vi "read burron.vi"() -> ()   [LabVIEW 2017]
panel:
  in  "GPIO":string(combo)
  out "LED indicator":string="LED OFF"
  out "button state":string="LED is turned on"
  out "error out 2":errorcluster
  in  "stop":bool
  out "error out":errorcluster
  in  "mode (standard)":T1(ring)
  in  "bytes to read":i32=1 min=1
  out "data out":string
  in  "Send Button":bool
  in  "Port":u16
  in  "address":string
  in  "data in":string
  out "bytes written":i32
  in  "stop 1":bool
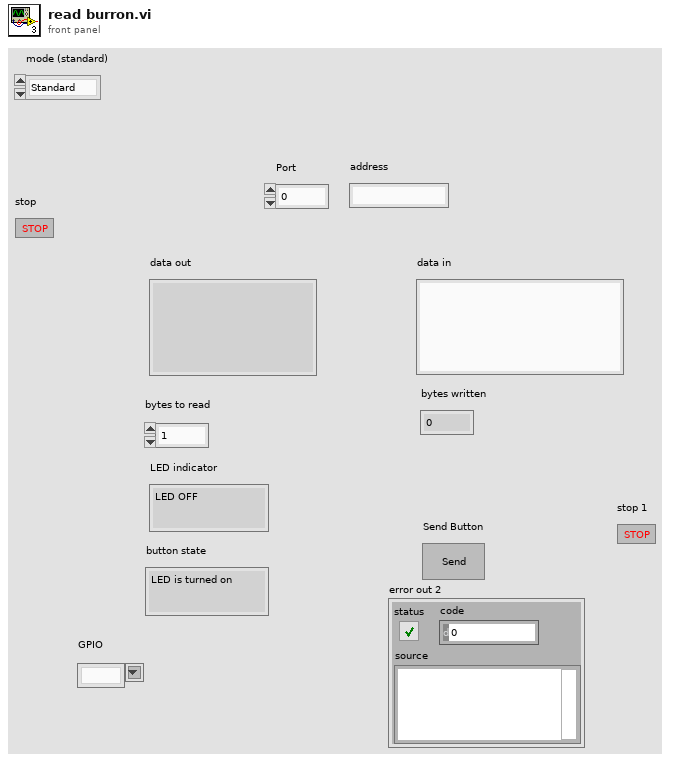
[diagram p1: front panel]
types:
  T1 = enum16{"Standard", "Buffered", "CRLF", "Immediate"}
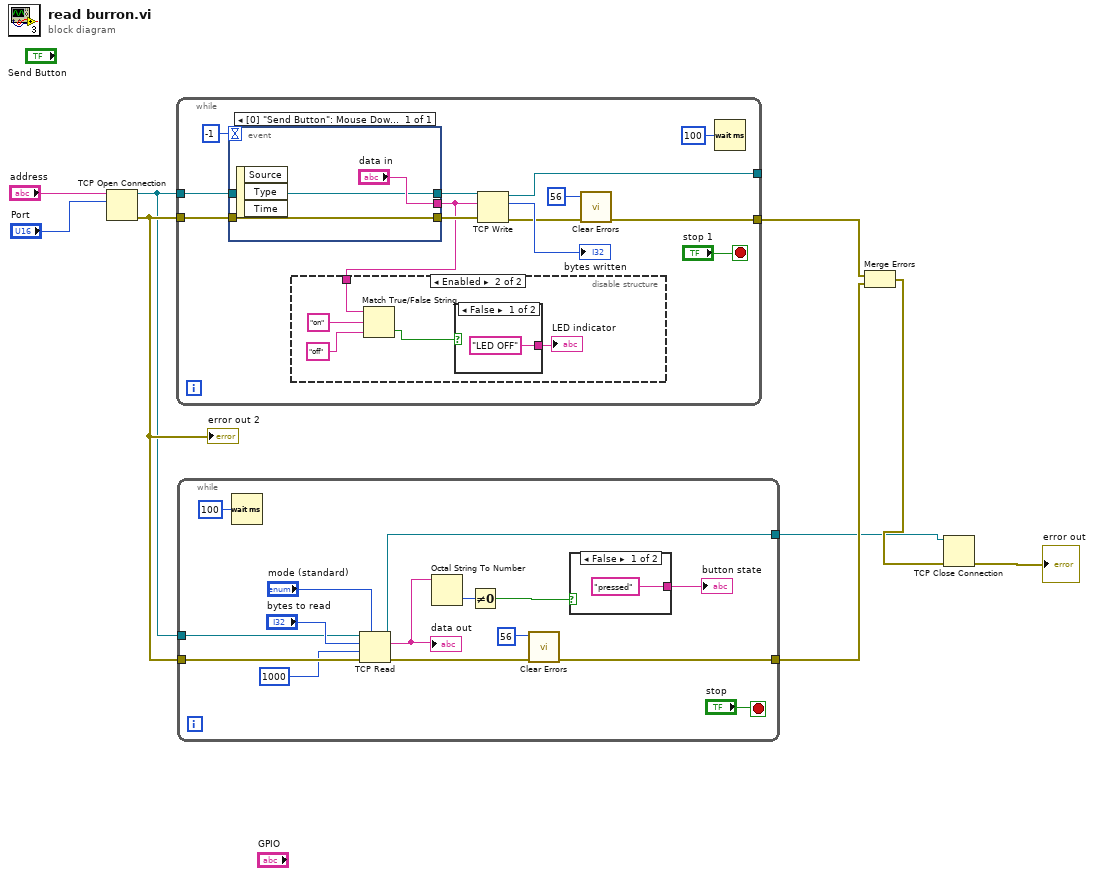
[diagram p0: block diagram]
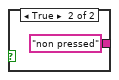
[diagram p2: hidden frame]
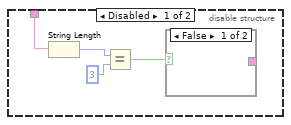
[diagram p3: hidden frame]
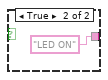
[diagram p4: hidden frame]
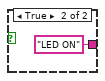
[diagram p5: hidden frame]
diagram:
  n1 = TCP Open Connection(address="address", remote port or service name="Port") -> (connection ID=w1:refnum<k5>, error out=w2:errorcluster)  [unwired: 3 in]
  "error out 2" <- w2
  n2 = while {
    tunnel: w1 -> [w12]
    tunnel: [w22] -> _
    tunnel: w2 -> [w15]
    tunnel: [w16] -> w7
    stop <- "stop 1" stop-if-true
    n3 = event shown="[0] \"Send Button\": Mouse Down;  Timeout" {
      selector: _ -> [_]
      dyn-events: _ -> [_]
      timeout: -1 -> [_]
      tunnel: ["data in"] -> w10
      tunnel: w15 -> [w36]
      tunnel: [w36] -> w14
      tunnel: [w35] -> w13
      tunnel: w12 -> [w35]
      event "Send Button": Mouse Down; Timeout {
        n4 = event-data() -> ()  [unwired: 1 in, 3 out]
      }
    }
    n5 = disable-structure shown="Enabled" {
      disable-tunnel: w10 -> [w26 w31]
      frame Disabled {
        n6 = String Length(string=w26) -> (length=w25:i32)
        n7 = Equal?(x=w25, y=3) -> (x = y?=w23:bool)
        n8 = case shown="False" w23 {
          tunnel: [_ "LED ON"] -> _
          frame False {
          }
          frame True {
          }
        }
      }
      frame Enabled {
        n9 = Match True/False String(2:"off" ("false string"), 3:"on" ("true string"), 4:w31) -> (0:w28:bool)  [unwired: 1 out]
        n10 = case shown="False" w28 {
          tunnel: ["LED OFF" "LED ON"] -> w32
          frame False {
          }
          frame True {
          }
        }
        "LED indicator" <- w32
      }
    }
    n11 = TCP Write(connection ID=w13, data in=w10, error in (no error)=w14) -> (connection ID out=w22:refnum<k5>, bytes written=→"bytes written":i32, error out=w17:errorcluster)  [unwired: 1 in]
    n12 = call <vilib>:"Clear Errors.vi"("error in (no error)"=w17, "specific error code to clear (0: all)"=56) -> ("error out"=w16:errorcluster)  [unwired: 4 in, 1 out]
    n13 = Wait (ms)(milliseconds to wait=u32 100) -> ()  [unwired: 1 out]
  }
  n14 = while {
    tunnel: [w48] -> w4
    tunnel: [w47] -> w3
    tunnel: w2 -> [w46]
    tunnel: w1 -> [w45]
    stop <- "stop" stop-if-true
    n15 = Wait (ms)(milliseconds to wait=u32 100) -> ()  [unwired: 1 out]
    n16 = TCP Read(connection ID=w45, bytes to read="bytes to read", error in (no error)=w46, 7:"mode (standard)", 9:1000 ("timeout ms (25000)")) -> (connection ID out=w47:refnum<k5>, data out=w39:string, error out=w51:errorcluster)
    "data out" <- w39
    n17 = Octal String To Number(4:w39) -> (0:w41:u32)  [unwired: 2 in, 1 out]
    n18 = Not Equal To 0?(x=w41) -> (x != 0?=w42:bool)
    n19 = call <vilib>:"Clear Errors.vi"("error in (no error)"=w51, "specific error code to clear (0: all)"=56) -> ("error out"=w48:errorcluster)  [unwired: 4 in, 1 out]
    n20 = case shown="False" w42 {
      tunnel: ["pressed" "non pressed"] -> w40
      frame False {
      }
      frame True {
      }
    }
    "button state" <- w40
  }
  n21 = Merge Errors(w7, w4) -> (w6:errorcluster)
  n22 = TCP Close Connection(connection ID=w3, error in (no error)=w6) -> (error out=→"error out":errorcluster)  [unwired: 1 in, 1 out]
